vi "LWXPS_MultipleAxesPVTExecution.vi"(0 "XPS Reference IN":refnum<k24>, 5 "Group Name":string, 7 "Trajectory File Name":string, 9 "Execution Number":i32, 11 "LabVIEW error IN":errorcluster) -> (4 "XPS Reference OUT":refnum<k24>, 6 "Returned error code":i32, 8 "XPS Error String":string, 15 "LabVIEW error OUT":errorcluster)   [LabVIEW 2014]
uses:
  D:/XPSQ8_LabView_Library/Development/Source/Dll/Newport.XPS.CommandInterface.dll
  Dll/Newport.XPS.CommandInterface.dll
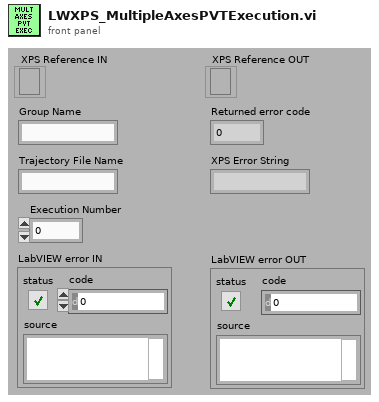
[diagram p1: front panel]
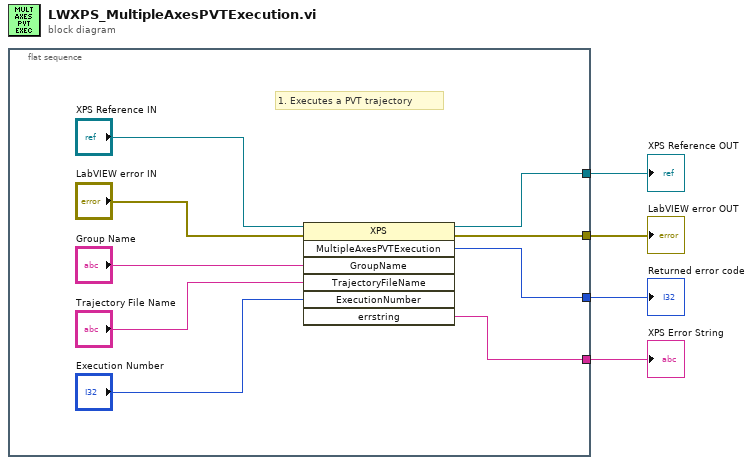
[diagram p0: block diagram]
diagram:
  n1 = flat-sequence {
    tunnel: [w11] -> w4
    tunnel: [w13] -> w3
    tunnel: [w10] -> w2
    tunnel: [w8] -> w1
    frame #0 {
      # "1. Executes a PVT trajectory"
      n2 = invoke class="XPS" method="MultipleAxesPVTExecution"(reference="XPS Reference IN", error in="LabVIEW error IN", "GroupName"="Group Name", "TrajectoryFileName"="Trajectory File Name", "ExecutionNumber"="Execution Number") -> (reference out=w11:refnum<k24>, error out=w13:errorcluster, "MultipleAxesPVTExecution"=w10:i32, "errstring"=w8:string)  [unwired: 2 in, 3 out]
    }
  }
  "XPS Reference OUT" <- w4
  "LabVIEW error OUT" <- w3
  "Returned error code" <- w2
  "XPS Error String" <- w1
